vi "Test_ListTables_WorksNoError.vi"(8 "error in (no error)":errorcluster, 11 "TestCase in":refnum<class "Test mysql.lvclass">) -> (0 "error out":errorcluster, 3 "TestCase out":refnum<class "Test mysql.lvclass">)   [LabVIEW 2020, in "DataBase_mysql_Tests.lvlib" / "Test mysql.lvclass"]
uses:
  Test mysql.lvclass
  externals/mysql/Source/mysql.net/mysql.lvclass
  <vilib>/addons/_JKI Toolkits/VI Tester/TestCase.llb/TestCase.lvclass
  C:/Program Files/National Instruments/LabVIEW 2020/vi.lib/addons/_JKI Toolkits/VI Tester/TestCase.llb/TestCase.lvclass
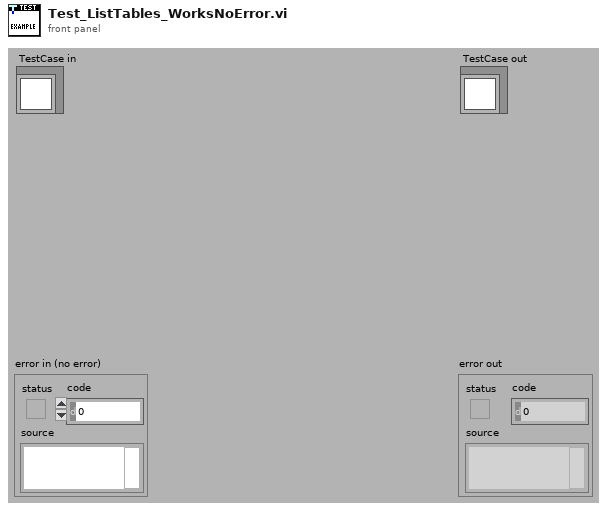
[diagram p1: front panel]
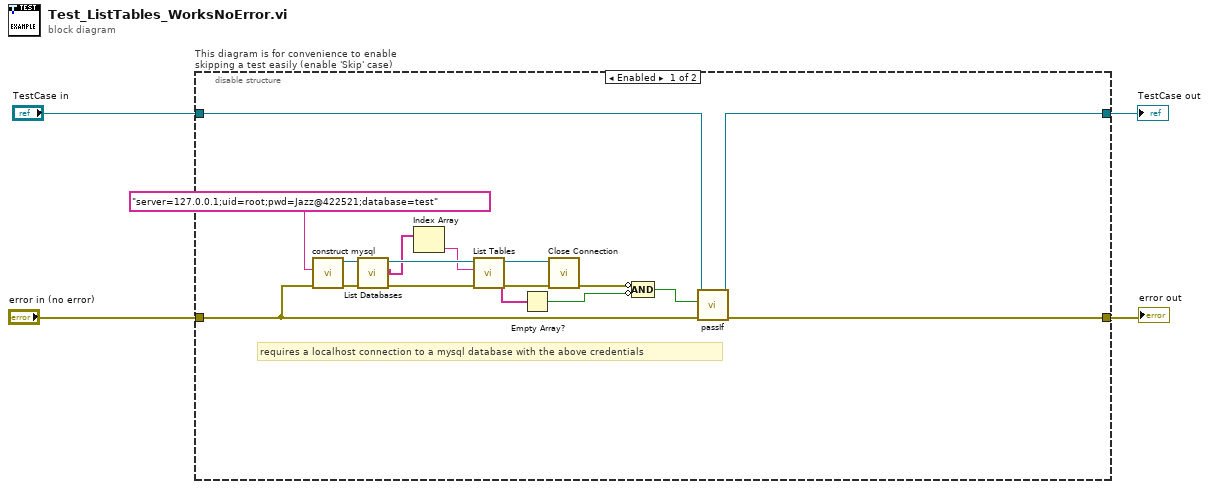
[diagram p0: block diagram]
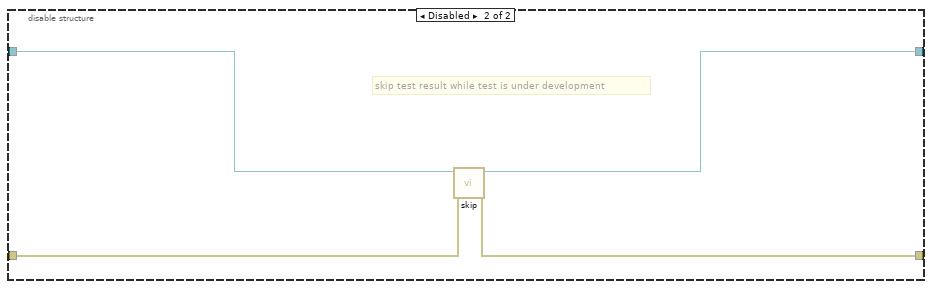
[diagram p2: hidden frame]
diagram:
  n1 = disable-structure "This diagram is for convenience to enable skipping a test easily (enable 'Skip' case)" shown="Enabled" {
    disable-tunnel: "TestCase in" -> [w21 w25]
    disable-tunnel: [w20 w23] -> w1
    disable-tunnel: [w19 w24] -> w3
    disable-tunnel: "error in (no error)" -> [w17 w22]
    frame Enabled {
      # "requires a localhost connection to a mysql database with the above credentials"
      n2 = call "construct mysql.vi"("error in (no error)"=w17, "Connection string"="server=127.0.0.1;uid=root;pwd=Jazz@422521;database=test") -> ("error out"=w10:errorcluster, "mysql out"=w9:refnum<class "mysql.lvclass">)  [unwired: 8 in]
      n3 = call-dynamic "List Databases.vi"("error in (no error)"=w10, "mysql in"=w9) -> ("error out"=w7:errorcluster, "databases"=w6:string[], "mysql out"=w8:refnum<class "mysql.lvclass">)  [unwired: 7 in]
      n4 = Index Array(array=w6) -> (element=w5:string)  [unwired: 1 in]
      n5 = call-dynamic "List Tables.vi"("error in (no error)"=w7, "database"=w5, "mysql in"=w8) -> ("error out"=w14:errorcluster, "tables"=w12:string[], "mysql out"=w13:refnum<class "mysql.lvclass">)  [unwired: 6 in]
      n6 = Empty Array?(array=w12) -> (empty?=w11:bool)
      n7 = call-dynamic "Close Connection.vi"("error in (no error)"=w14, "mysql in"=w13) -> ("error out"=w16:errorcluster)  [unwired: 8 in, 1 out]
      n8 = Compound Arithmetic op=AND(invert w16, invert w11) -> (w15:bool)
      n9 = call-dynamic "passIf.vi"("error in (no error)"=w17, "pass"=w15, "TestCase in"=w21) -> ("error out"=w19:errorcluster, "TestCase out"=w20:refnum<class "Test mysql.lvclass">)  [unwired: 7 in]
    }
    frame Disabled {
      # "skip test result while test is under development"
      n10 = call <vilib>:"skip.vi"("error in (no error)"=w22, "TestCase in"=w25) -> ("error out"=w24:errorcluster, "TestCase out"=w23:refnum<class "Test mysql.lvclass">)  [unwired: 8 in]
    }
  }
  "error out" <- w3
  "TestCase out" <- w1
